vi "SinewaveSiggen_USRPTx.vi"() -> ()   [LabVIEW 2021]
uses:
  system stop.vi
  <instrlib>/niUSRP/niUSRP Write Tx Data (CDB Cluster).vi
panel:
  in  "Tab Control":enum32{"SDR Settings", "Tx Waveform"}(tab)
  in  "IQ rate Tx":dbl=400000.0 format="%#_6p"
  in  "carrier frequency Tx":dbl=2400000000.0 format="%#_6p"
  in  "Tx Gain":dbl format="%#_6f"
  in  "Tx IP":refnum<k15>="192.168.10.2"
  out "coerced IQ rate Tx":dbl=100000.0 format="%#_6p"
  out "coerced carrier frequency Tx":dbl=100000.0 format="%#_6p"
  in  "Frequency":dbl=10000.0 format="%#_13g"
  in  "Duration":dbl=0.01 format="%#_13g"
  in  "Frequency 2":dbl=10000.0 format="%#_13g"
  out "Waveform Graph":dbl[](graph)
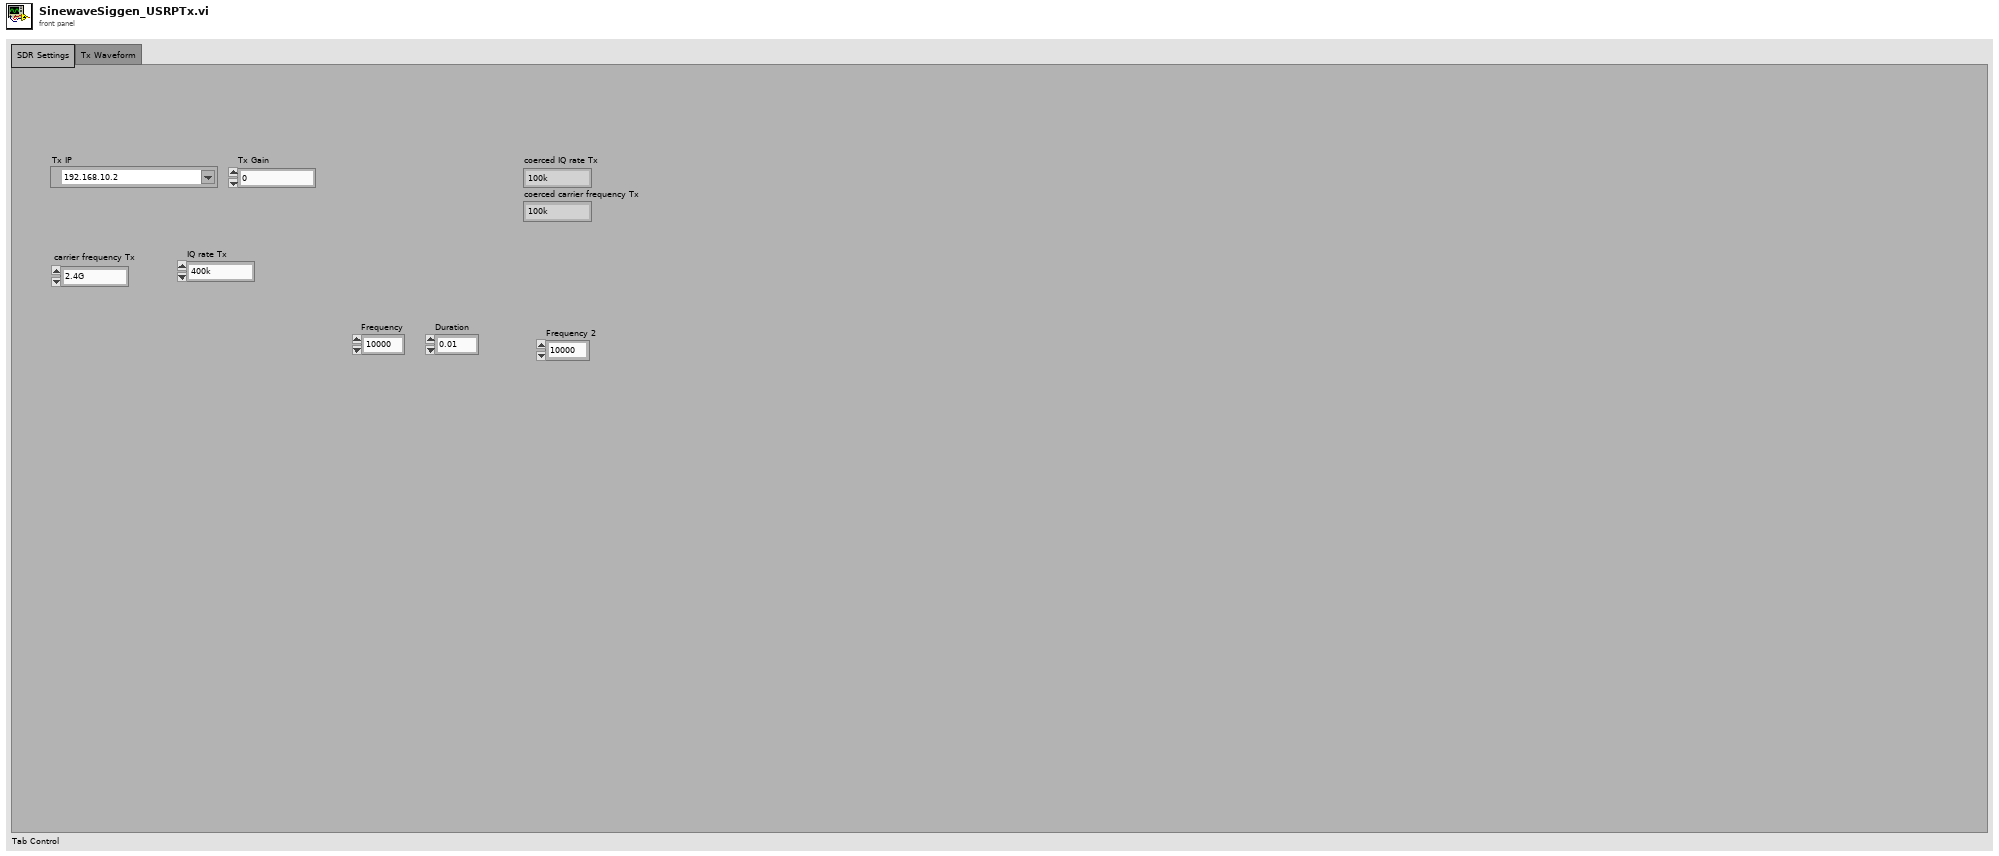
[diagram p1: front panel]
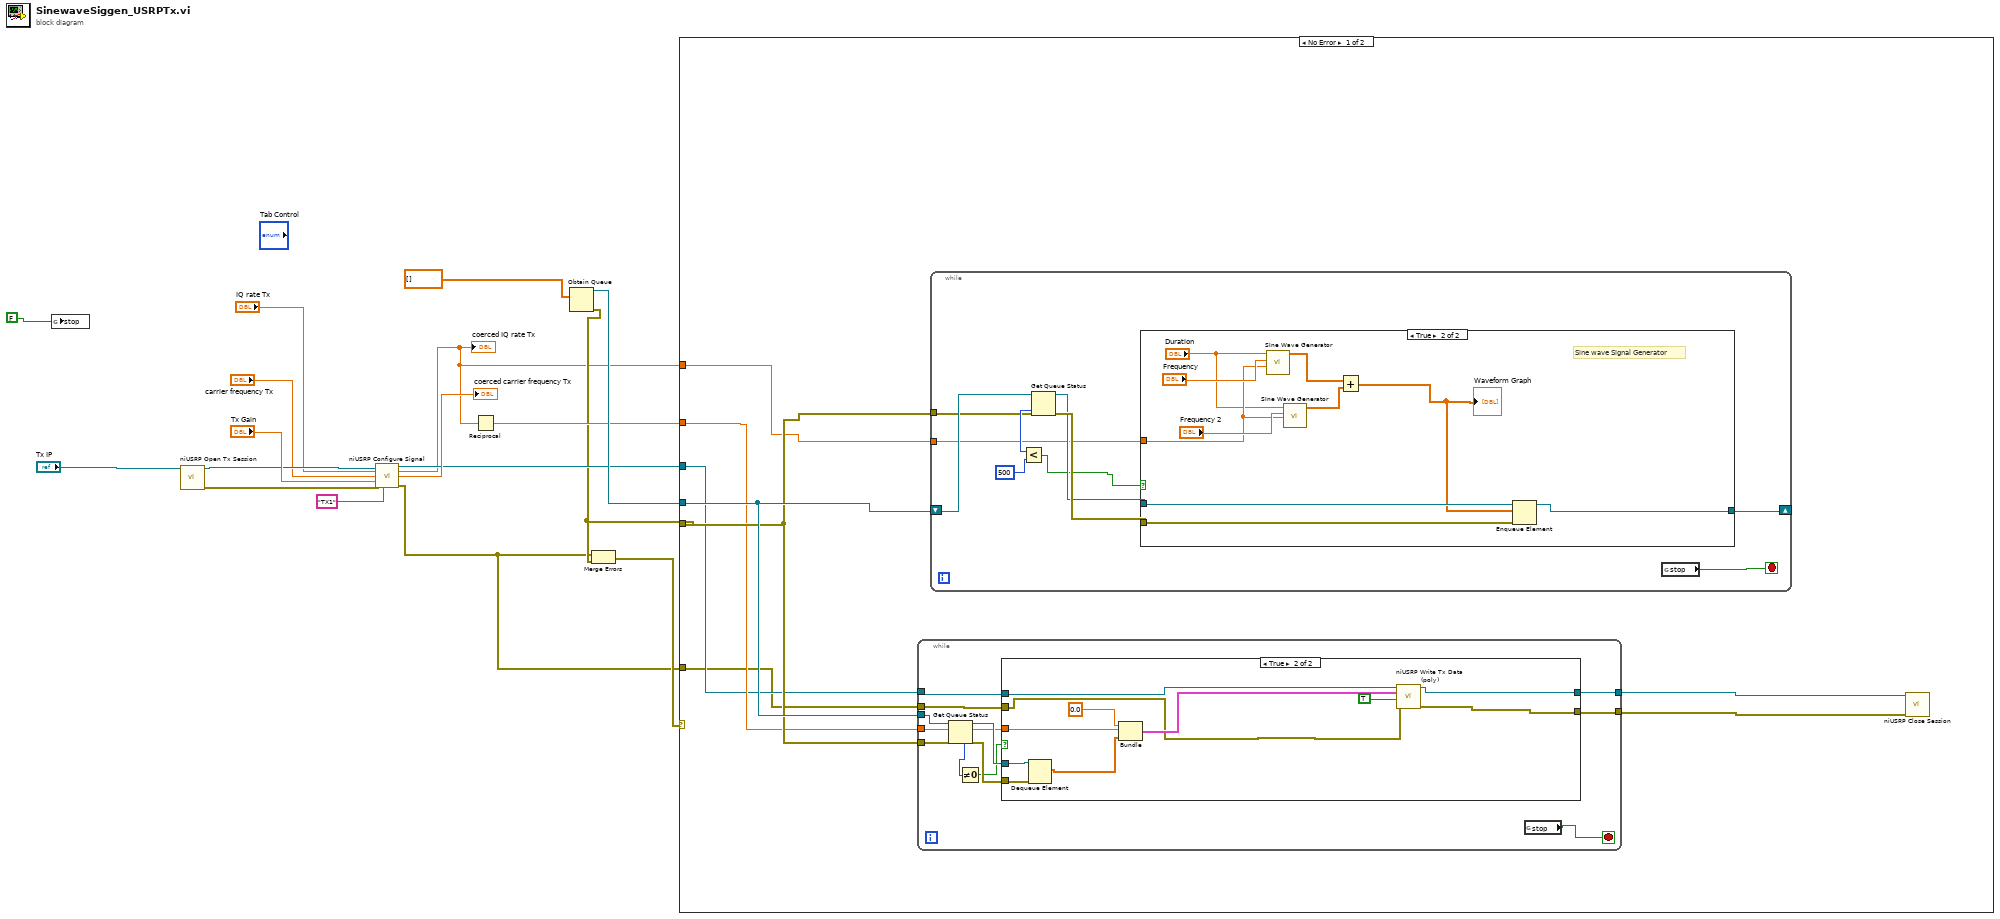
[diagram p0: block diagram]
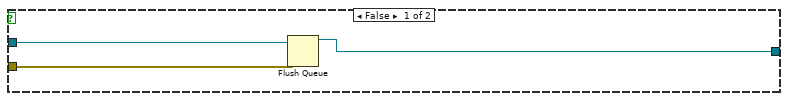
[diagram p2: hidden frame]
diagram:
  n1 = global write "system stop.vi" "stop"(FALSE) -> ()
  n2 = call <instrlib>:"niUSRP Open Tx Session.vi"("device names"="Tx IP") -> ("session handle out"=w15:refnum<k15>, "error out"=w14:errorcluster)  [unwired: 13 in]
  n3 = call <instrlib>:"niUSRP Configure Signal.vi"("session handle"=w15, "IQ rate"="IQ rate Tx", "carrier frequency"="carrier frequency Tx", "gain"="Tx Gain", "error in (no error)"=w14, "active antenna"="TX1") -> ("session handle out"=w8:refnum<k15>, "coerced IQ rate"=w5:dbl, "coerced carrier frequency"=→"coerced carrier frequency Tx":dbl, "error out"=w4:errorcluster)  [unwired: 5 in, 1 out]
  "coerced IQ rate Tx" <- w5
  n4 = Reciprocal(x=w5) -> (1/x=w7:dbl)
  n5 = Obtain Queue(element data type=dbl[] []) -> (queue out=w9:refnum<queue>, error out=w6:errorcluster)  [unwired: 4 in, 1 out]
  n6 = Merge Errors(w4, w6) -> (w11:errorcluster)
  n7 = case shown="No Error" w11 {
    tunnel: w6 -> [w24 _]
    tunnel: w9 -> [w25 _]
    tunnel: w8 -> [w22 _]
    tunnel: w7 -> [w23 _]
    tunnel: w5 -> [w21 _]
    tunnel: w4 -> [w20 _]
    frame No Error {
      n8 = while {
        tunnel: w25 -> [w60]
        tunnel: w24 -> [w57]
        tunnel: w23 -> [w56]
        tunnel: w22 -> [w54]
        tunnel: w20 -> [w52]
        tunnel: [w50] -> w19
        tunnel: [w49] -> w18
        stop <- w51 stop-if-true
        n9 = Get Queue Status(queue=w60, error in (no error)=w57) -> (queue out=w59:refnum<queue>, error out=w58:errorcluster, # elements in queue=w55:i32)  [unwired: 1 in, 5 out]
        n10 = Not Equal To 0?(x=w55) -> (x != 0?=w53:bool)
        n11 = case shown="True" w53 {
          tunnel: w59 -> [_ w73]
          tunnel: w58 -> [_ w72]
          tunnel: w56 -> [_ w71]
          tunnel: w54 -> [w62 w69]
          tunnel: w52 -> [w61 w63]
          tunnel: [w62 w65] -> w50
          tunnel: [w61 w64] -> w49
          frame False {
          }
          frame True {
            n12 = Dequeue Element(queue=w73, error in (no error)=w72) -> (element=w68:dbl[])  [unwired: 1 in, 3 out]
            n13 = Bundle(0.0, w71, w68) -> (w70:cluster{dbl, dbl, dbl[]})  [unwired: 1 in]
            n14 = call-poly <instrlib>:"niUSRP Write Tx Data (poly).vi"("session handle"=w69, "data"=w70, "end of data?"=TRUE, "error in (no error)"=w63) -> ("session handle out"=w65:refnum<k15>, "error out"=w64:errorcluster)  [unwired: 10 in]
          }
        }
        n15 = global read "system stop.vi" "stop"() -> (w51:bool)
      }
      n16 = while {
        tunnel: w24 -> [w30]
        tunnel: w21 -> [w29]
        shift-right: [w28] -> _
        shift-left: w25 -> [w31]
        stop <- w27 stop-if-true
        n17 = Get Queue Status(queue=w31, error in (no error)=w30) -> (queue out=w32:refnum<queue>, error out=w33:errorcluster, # elements in queue=w35:i32)  [unwired: 1 in, 5 out]
        n18 = Less?(x=w35, y=500) -> (x < y?=w26:bool)
        n19 = case shown="True" w26 {
          tunnel: w33 -> [w37 w48]
          tunnel: w32 -> [w38 w47]
          tunnel: w29 -> [_ w43]
          tunnel: [w36 w45] -> w28
          frame False {
            n20 = Flush Queue(queue=w38, error in (no error)=w37) -> (queue out=w36:refnum<queue>)  [unwired: 2 out]
          }
          frame True {
            # "Sine wave Signal Generator"
            n21 = call "SIne Wave Generator.vi"("Sampling rate"=w43, "Frequency"="Frequency", "Duration"="Duration") -> ("Array"=w41:dbl[])  [unwired: 7 in, 1 out]
            n22 = call "SIne Wave Generator.vi"("Sampling rate"=w43, "Frequency"="Frequency 2", "Duration"="Duration") -> ("Array"=w40:dbl[])  [unwired: 7 in, 1 out]
            n23 = Add(x=w41, y=w40) -> (x+y=w39:dbl[])
            "Waveform Graph" <- w39
            n24 = Enqueue Element(queue=w47, element=w39, error in (no error)=w48) -> (queue out=w45:refnum<queue>)  [unwired: 1 in, 2 out]
          }
        }
        n25 = global read "system stop.vi" "stop"() -> (w27:bool)
      }
      n26 = call <instrlib>:"niUSRP Close Session.vi"("session handle"=w19, "error in (no error)"=w18) -> ()  [unwired: 13 in, 1 out]
    }
    frame Error {
    }
  }
